vi "Prototype.vi"() -> ()   [LabVIEW 2013, in "J1939 tests.lvlib"]
uses:
  module/configuration/XNET Settings.ctl
  module/configuration/J1939 configuration.lvclass
  module/configuration/J1939 configuration.lvclass/J1939 configuration.ctl
  module/configuration/Write XNET Settings.vi
  module/configuration/Read XNET Settings.vi
  <vilib>/xnet/xnet.llb/XNET Create Session (Signal Input Single-point).vi
  Program Files (x86)/National Instruments/LabVIEW 2013/examples/nixnet/examples.llb/NI-XNET Example subVI - J1939 Claim With Address.vi
  <vilib>/xnet/xnet.llb/XNET Create Session (Signal Output Single-point).vi
  <vilib>/xnet/xnet.llb/XNET Write (Signal Single-point).vi
  <vilib>/xnet/xnet.llb/XNET Read (Signal Single-point).vi
  J1939 tests.lvlib
panel:
  in  "Array":refnum<k21>[](array[refnum])=["Aftertreatment1SecondAirPress\nj1939", "AmbientAirTemp\nj1939", "BrakeTemperature\nj1939", "PowerTakeoffOilTemp\nj1939"]
  in  "Write 2":bool
  in  "XNET Settings 2":T1={"Select Interface"="CAN1", "Node Address"=1, "Node Name"=1}
  in  "XNET Settings":T1={"Select Interface"="CAN2", "Node Address"=1, "Node Name"=1}
  in  "Signal Single Point Data 2":dbl[](array[knob])=[0.0, 0.0] caption="data" scale=0.0..50.0
  in  "stop":bool
  out "Signal Single Point Data":dbl[](array[knob]) caption="data" scale=0.0..50.0
  in  "Update":bool
  out "Select Signal List from database":refnum<k21>[](array[refnum])=["J1939_LargeSignal1\nNIXNET_example.J1939_Over_CAN", "J1939_LargeSignal2\nNIXNET_example.J1939_Over_CAN"]
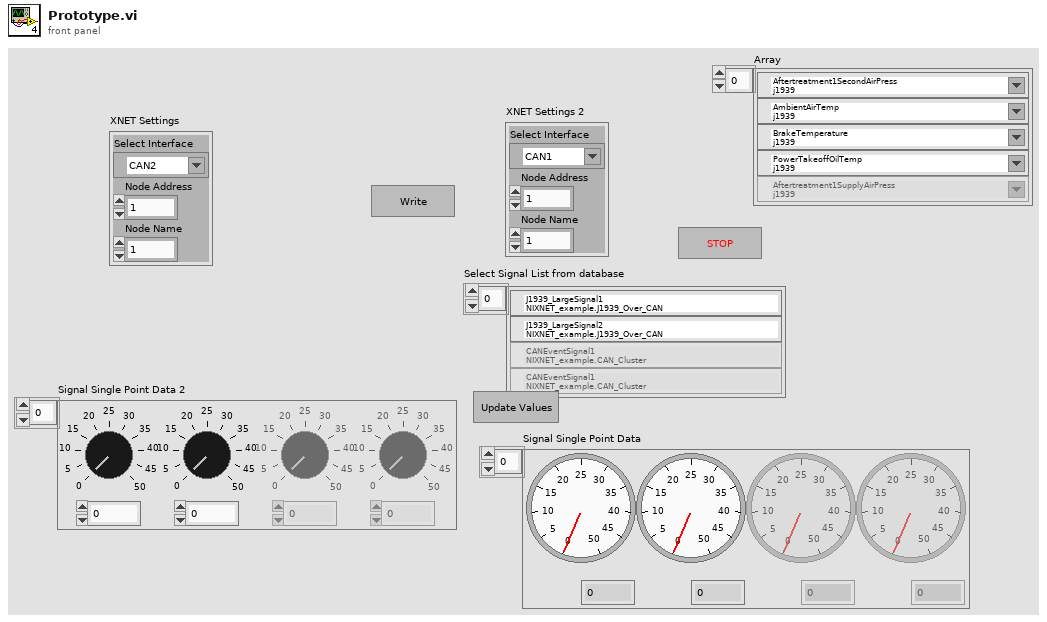
[diagram p1: front panel]
types:
  T1 = typedef "J1939 configuration.lvclass/XNET Settings.ctl" = cluster{"Select Interface":refnum<k21>, "Node Address":u8, "Node Name":u64}
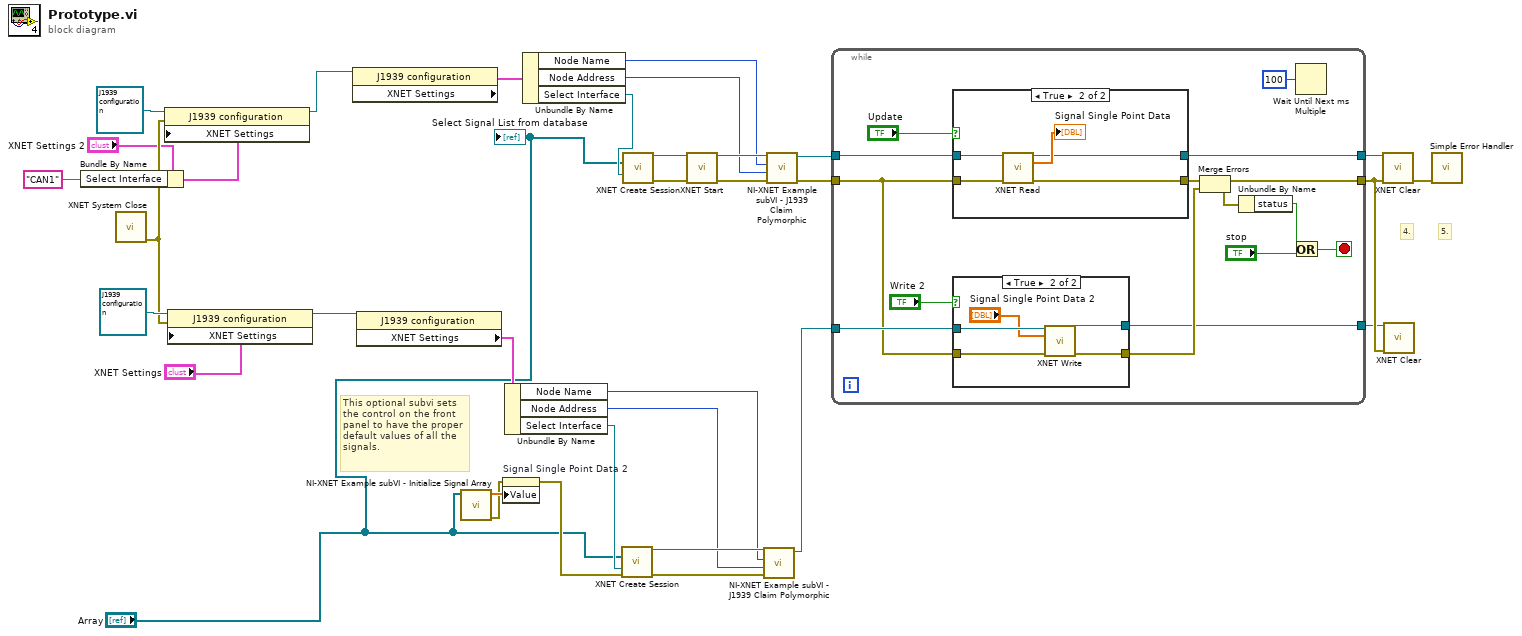
[diagram p0: block diagram]
diagram:
  # "This optional subvi sets the control on the front panel to have the proper default values of all the signals."
  # "5."
  # "4."
  n1 = Bundle By Name(cluster="XNET Settings 2", "Select Interface"="CAN1") -> (w2:T1)
  n2 = call <vilib>:"XNET System Close.vi"() -> ("error out"=w5:errorcluster)  [unwired: 15 in]
  n3 = property class="J1939 configuration"(reference=refnum<class "J1939 configuration.lvclass"> refnum ("J1939 configuration"), error in=w5, "XNET Settings"=w2) -> (reference out=w18:refnum<class "J1939 configuration.lvclass">)  [unwired: 1 out]
  n4 = property class="J1939 configuration"(reference=refnum<class "J1939 configuration.lvclass"> refnum ("J1939 configuration"), error in=w5, "XNET Settings"="XNET Settings") -> (reference out=w17:refnum<class "J1939 configuration.lvclass">)  [unwired: 1 out]
  n5 = property class="J1939 configuration"(reference=w18) -> ("XNET Settings"=w12:T1)  [unwired: 1 in, 2 out]
  n6 = property class="J1939 configuration"(reference=w17) -> ("XNET Settings"=w16:T1)  [unwired: 1 in, 2 out]
  n7 = call "NI-XNET Example subVI - Initialize Signal Array.vi"("signal list"="Array") -> ("error out"=w25:errorcluster, "Array"=w26:dbl[])  [unwired: 1 in, 6 out]
  n8 = property on="Signal Single Point Data 2" class="Arr (strict)"(error in=w25, "Value"=w26) -> (error out=w24:errorcluster)  [unwired: 1 in, 1 out]
  n9 = Unbundle By Name(w16) -> ("Node Name"=w15:u64, "Node Address"=w14:u8, "Select Interface"=w13:refnum<k21>)
  n10 = Unbundle By Name(w12) -> ("Node Name"=w10:u64, "Node Address"=w11:u8, "Select Interface"=w9:refnum<k21>)
  n11 = call-poly <vilib>:"XNET Create Session.vi"("signal list"="Array", "interface"=w13, "error in (no error)"=w24) -> ("session out"=w23:refnum<k21>, "error out"=w22:errorcluster)  [unwired: 11 out]
  n12 = call-poly <vilib>:"XNET Create Session.vi"("signal list"="Array", "interface"=w9) -> ("session out"=w34:refnum<k21>, "error out"=w33:errorcluster)  [unwired: 1 in, 11 out]
  n13 = call <vilib>:"XNET Start.vi"("session in"=w34, "error in (no error)"=w33) -> ("session out"=w30:refnum<k21>, "error out"=w29:errorcluster)  [unwired: 12 in]
  n14 = call-poly "NI-XNET Example subVI - J1939 Claim Polymorphic.vi"("error in (no error)"=w22, "SAE J1939:Node Address"=w14, "SAE J1939:Node Name"=w15, "XNET Session"=w23) -> ("XNET Session Out"=w8:refnum<k21>)  [unwired: 5 in, 2 out]
  n15 = call-poly "NI-XNET Example subVI - J1939 Claim Polymorphic.vi"("error in (no error)"=w29, "SAE J1939:Node Address"=w11, "SAE J1939:Node Name"=w10, "XNET Session"=w30) -> ("error out"=w28:errorcluster, "XNET Session Out"=w27:refnum<k21>)  [unwired: 5 in, 1 out]
  n16 = while {
    tunnel: [w36] -> w7
    tunnel: w27 -> [w45]
    tunnel: w28 -> [w39]
    tunnel: [w42] -> w31
    tunnel: w8 -> [w40]
    tunnel: [w35] -> w6
    stop <- w46 stop-if-true
    n17 = case shown="True" "Update" {
      tunnel: [w57 w62] -> w37
      tunnel: w45 -> [w56 w60]
      tunnel: w39 -> [w57 w59]
      tunnel: [w56 w58] -> w42
      frame False {
      }
      frame True {
        n18 = call-poly <vilib>:"XNET Read.vi"("session in"=w60, "error in (no error)"=w59) -> ("session out"=w58:refnum<k21>, "data"=→"Signal Single Point Data":dbl[], "error out"=w62:errorcluster)  [unwired: 11 out]
      }
    }
    n19 = case shown="True" "Write 2" {
      tunnel: w40 -> [w49 w55]
      tunnel: w39 -> [w50 w54]
      tunnel: [w50 w53] -> w38
      tunnel: [w49 w51] -> w35
      frame False {
      }
      frame True {
        n20 = call-poly <vilib>:"XNET Write.vi"("session in"=w55, "data"="Signal Single Point Data 2", "error in (no error)"=w54) -> ("session out"=w51:refnum<k21>, "error out"=w53:errorcluster)  [unwired: 11 out]
      }
    }
    n21 = Merge Errors(w37, w38) -> (w36:errorcluster)
    n22 = Unbundle By Name(w36) -> ("status"=w48:bool)
    n23 = Or(x=w48, y="stop") -> (x .or. y?=w46:bool)
    n24 = Wait Until Next ms Multiple(millisecond multiple=u32 100 ("milliseconds to wait")) -> ()  [unwired: 1 out]
  }
  n25 = call <vilib>:"XNET Clear.vi"("session in"=w31, "error in (no error)"=w7) -> ("error out"=w32:errorcluster)  [unwired: 13 in]
  n26 = call <vilib>:"XNET Clear.vi"("session in"=w6, "error in (no error)"=w7) -> ()  [unwired: 13 in, 1 out]
  n27 = call <vilib>:"Simple Error Handler.vi"("error in (no error)"=w32) -> ()  [unwired: 1 in, 8 out]
  "Select Signal List from database" <- "Array"
